vi "displaySummaryState.vi"(10 "viewThisComponent":refnum<class "ViewThisComponent.lvclass">) -> ()   [LabVIEW 2016, in "EXAViewElements.lvlib"]
doc: "Displays summary state information."
uses:
  EXAViewElements.lvlib
  ComponentTemplateCore/GUI/SummaryStateIndicator/SummaryStatePictRing.ctl
  ViewThisComponent/ViewThisComponent.lvclass
  home/andres/ct_cmpuserevents/ComponentTemplateCore/ComponentModel/ComponentModel/View/View.lvclass
  ComponentTemplateCore/ComponentModel/ComponentModel/View/View.lvclass
panel:
  out "EXA:":T1
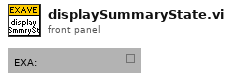
[diagram p1: front panel]
types:
  T1 = typedef "SummaryStatePictRing.ctl" = u16
  T2 = typedef "EXATypedefs.lvlib/PubDataEvents.ctl" = cluster{"DetailedState":refnum<user-event>, "ErrorCode":refnum<user-event>, "Heartbeat":refnum<user-event>, "LoopTime_ms":refnum<user-event>, "LoopTimeOutOfRange":refnum<user-event>, "RejectedCommand":refnum<user-event>, "Timestamp":refnum<user-event>, "AppliedSettingsMatchStart":refnum<user-event>, "SettingsApplied":refnum<user-event>, "SettingVersions":refnum<user-event>, "SummaryState":refnum<user-event>}
  T3 = enum16{"", " ENABLED", " DISABLED", " STANDBY", " OFFLINE", " FAULT"}
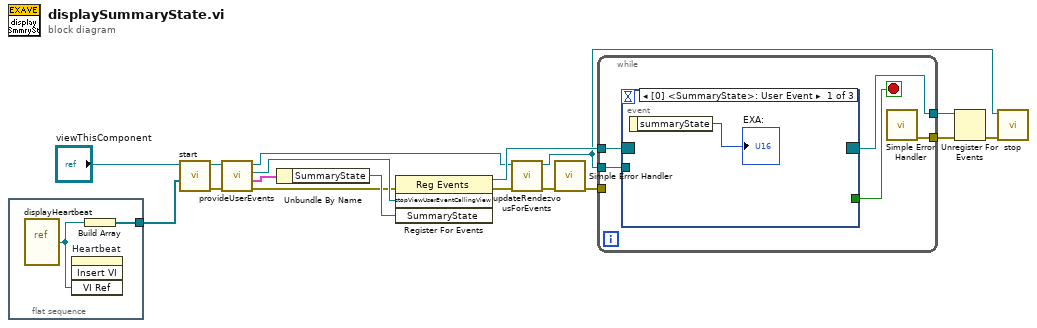
[diagram p0: block diagram]
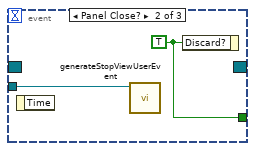
[diagram p2: hidden frame]
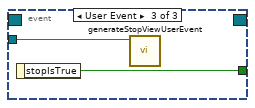
[diagram p3: hidden frame]
diagram:
  n1 = flat-sequence {
    tunnel: [w19] -> w17
    frame #0 {
      n2 = vi-ref "displayHeartbeat.vi"() -> (w18:refnum<vi>)
      n3 = invoke on="Heartbeat" class="SubPnl" method="Insert VI"("VI Ref"=w18) -> ()  [unwired: 3 in, 4 out]
      n4 = Build Array(w18) -> (w19:refnum<vi>[])
    }
  }
  n5 = call-dynamic "start.vi"("subpanelVIRefs"=w17, "View in"="viewThisComponent") -> ("error out"=w11:errorcluster, "View out"=w12:refnum<class "ViewThisComponent.lvclass">)  [unwired: 8 in]
  n6 = call "provideUserEvents.vi"("error in (no error)"=w11, "ViewThisComponent in"=w12) -> ("error out"=w10:errorcluster, "pubDataEvents"=w13:T2, "stopViewUserEventCallingView"=w14:refnum<user-event>, "ViewThisComponent out"=w4:refnum<class "ViewThisComponent.lvclass">)  [unwired: 6 in]
  n7 = Unbundle By Name(w13) -> ("SummaryState"=w15:refnum<user-event>)
  n8 = register-events(error in=w10, w14, w15) -> (reference out=w9:refnum<event-registration>, error out=w2:errorcluster)  [unwired: 1 in]
  n9 = call "updateRendezvousForEvents.vi"("error in (no error)"=w2, "View in"=w4) -> ("error out"=w1:errorcluster, "View out"=w3:refnum<class "ViewThisComponent.lvclass">)  [unwired: 8 in]
  n10 = call <vilib>:"Simple Error Handler.vi"("error in (no error)"=w1) -> ("error out"=w5:errorcluster)  [unwired: 4 in, 4 out]
  n11 = while {
    tunnel: w9 -> [w24]
    tunnel: w3 -> [w23]
    tunnel: [w21] -> w8
    tunnel: [w20] -> w6
    tunnel: w5 -> [_]
    stop <- w22 stop-if-true
    n12 = event shown="[0] <SummaryState>: User Event" {
      selector: w24 -> [_ _ _]
      dyn-events: [_ _ _] -> w21
      timeout: _ -> [_ _ _]
      tunnel: w23 -> [_ w27 w28]
      tunnel: [_ w26 w29] -> w22
      event User Event {
        n13 = event-data() -> ("summaryState"=→"EXA:":T3)  [unwired: 1 in]
      }
      event Panel Close? {
        w26 = TRUE
        n14 = event-data() -> ()  [unwired: 1 in, 1 out]
        n15 = call "generateStopViewUserEvent.vi"("View in"=w27) -> ()  [unwired: 9 in, 2 out]
        n16 = event-data("Discard?"=w26) -> ()  [unwired: 1 in, 1 out]
      }
      event User Event {
        n17 = event-data() -> ("stopIsTrue"=w29:bool)  [unwired: 1 in]
        n18 = call "generateStopViewUserEvent.vi"("View in"=w28) -> ()  [unwired: 9 in, 2 out]
      }
    }
    n19 = call <vilib>:"Simple Error Handler.vi"() -> ("error out"=w20:errorcluster)  [unwired: 5 in, 4 out]
  }
  n20 = Unregister For Events(event registration refnum=w8, error in=w6) -> (error out=w7:errorcluster)
  n21 = call-dynamic "stop.vi"("error in (no error)"=w7, "View in"=w3) -> ()  [unwired: 8 in, 2 out]
